vi "aquire data.vi"(11 "Template in":refnum<class "Template.lvclass">) -> (0 "error out":errorcluster, 3 "Template out":refnum<class "Template.lvclass">)   [LabVIEW 2020, in "Template.lvlib" / "Template.lvclass"]
doc: "Executes the data acquisition routine defined by the hardware.\nUse the provided APIs to tap into this actor's queues reference by using the Read Actor Queues.vi or your own inside the child class private data.\n\n<b> Pack the data as follows</b>\n\n<b>- Header:</b> array of 145 bytes comprised of\n - Priority: 1 byte (0: Act immediately and report errors, 1: Act immediately but disregard errors, 2: Do not process)\n - Timestamp: 16 bytes\n - Metadata: Reserved for specific use, 128 bytes\n<b>- Data:</b> Variable size bite array\n<b>- Footer:</b> Reserved for specific use, 128 bytes"
uses:
  Template.lvclass
  Template.lvclass/Template.ctl
  <vilib>/numeric/Random Number (Range) U64.vi
  <vilib>/numeric/sub_Random U32.vi
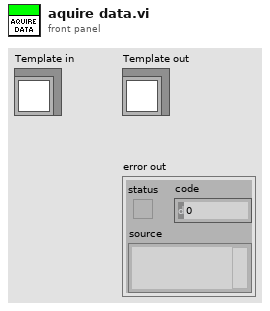
[diagram p1: front panel]
types:
  T1 = typedef "Template.lvlib/Template.lvclass/base actor queues.ctl" = cluster{"DVR Pool":refnum<queue>, "Actor's Data":refnum<queue>}
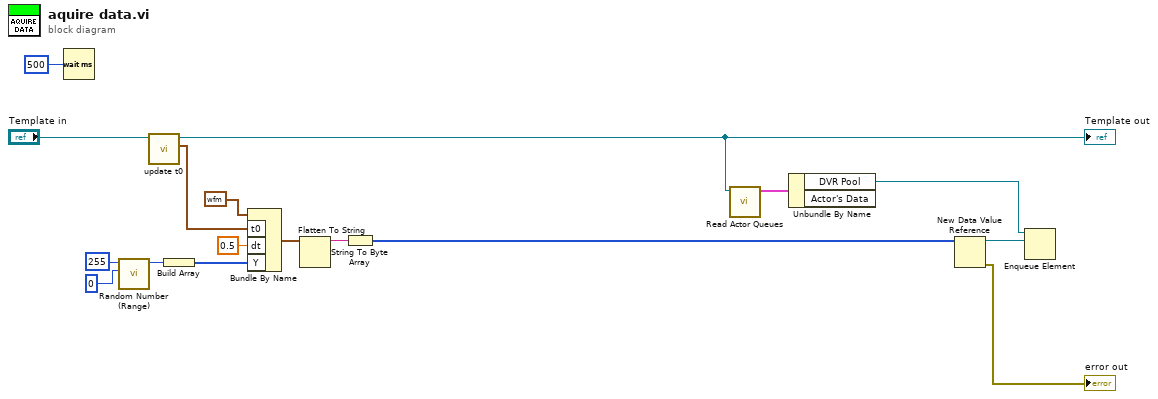
[diagram p0: block diagram]
diagram:
  n1 = Wait (ms)(milliseconds to wait=u32 500) -> ()  [unwired: 1 out]
  n2 = call-poly <vilib>:"Random Number (Range).vi"("lower bound (0)"=u64 0, "upper bound (100)"=u64 255) -> ("number"=w16:u64)  [unwired: 9 in]
  n3 = call "update t0.vi"("Template in"="Template in") -> ("t0"=w6:timestamp, "Template out"=w7:refnum<class "Template.lvclass">)  [unwired: 9 in]
  "Template out" <- w7
  n4 = Build Array(w16) -> (w15:u64[])
  n5 = Bundle By Name(cluster=waveform(dbl) {"t0"=timestamp(0 s since 1904-01-01), "dt"=1.0, "Y"=[]} ("Waveform"), "t0"=w6, "dt"=0.5, "Y"=w15) -> (w5:waveform(dbl))
  n6 = Flatten To String(anything=w5) -> (data string=w4:string)  [unwired: 3 in, 2 out]
  n7 = String To Byte Array(string=w4) -> (unsigned byte array=w3:u8[])
  n8 = call "Read Actor Queues.vi"("Template in"=w7) -> ("Base Actor Queues"=w11:T1)  [unwired: 10 in]
  n9 = Unbundle By Name(w11) -> ("DVR Pool"=w10:refnum<queue>)  [unwired: 1 out]
  n10 = New Data Value Reference(data value=w3) -> (data value reference=w9:refnum<data-value>, error out=→"error out":errorcluster)  [unwired: 1 in]
  n11 = Enqueue Element(queue=w10, element=w9) -> ()  [unwired: 2 in, 3 out]
